vi "OutputSwerveAzimuth.vi"() -> ()   [LabVIEW 2020]
doc: "This VI runs feedback and feedforward controllers, manages safety interlocks, and sends commands to the swerve azimuth motors."
uses:
  robotoutputs.vi
  sensordata.vi
  TAI_Motor.vi
  <vilib>/Rock Robotics/WPI/ThirdParty/Phoenix-LabVIEW/Motor Controller/Controls/CTRE_Phoenix_MotorControl_ControlMode.ctl
  driverdata.vi
  <vilib>/Rock Robotics/WPI/ThirdParty/Phoenix-LabVIEW/Motor Controller/Controls/CTRE_Phoenix_MotorControl_NeutralMode.ctl
  6e813111-160f-47d9-be7e-04f12fb0a952.vi
  GRNF_CTREMotor.vi
  <vilib>/Rock Robotics/WPI/ThirdParty/Phoenix-LabVIEW/Motor Controller/Get/CTRE_Phoenix_MotorController_GetSelectedSensorData.vi
  GlobalDrivebase.vi
panel:
  in  "Slew Rate When Slow (/s)":dbl=50000.0
  in  "Slew Rate When Fast (/s)":dbl=5000.0
  out "Azimuth Error (deg)":dbl
  out "Azimuth Velocity":cluster{dbl}(graph)
  out "Azimuth Position":cluster{dbl, "Interlock Output":dbl}(graph)
  in  "PID Parameters":T1={"Kp"=0.3, "Ki"=0.0, "Kd"=0.0, "Kf (don't use)"=0.0, "I-Zone"=10.0} {"Kd" min=0.0; "Ki" min=0.0; "Kp" min=0.0}
  in  "Manual Azimuth Goal (deg) [-180,180]":dbl step=5.0
  in  "Manually Override Azimuth Goal":bool
  in  "Best Angle Hysteresis (deg)":dbl=20.0 format="%#_13g"
  in  "Plotting":T2(ring)
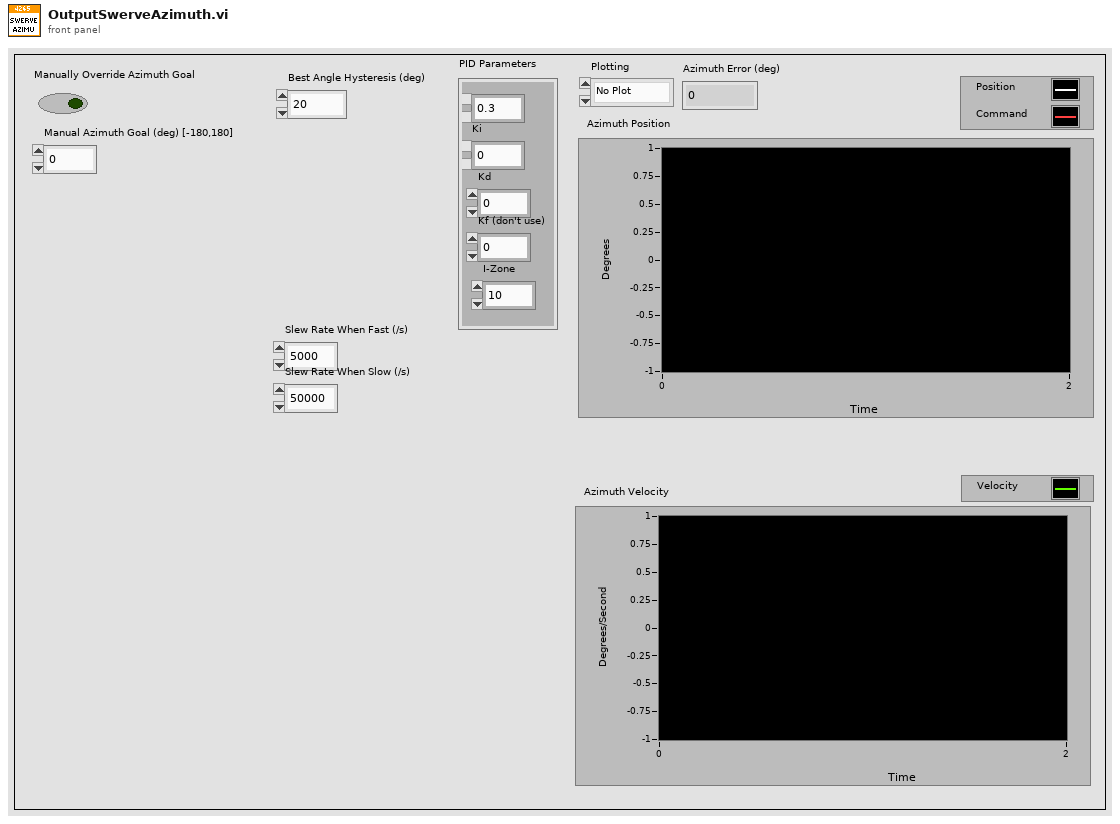
[diagram p1: front panel]
types:
  T1 = cluster{"Kp":dbl, "Ki":dbl, "Kd":dbl, "Kf (don't use)":dbl, "I-Zone":dbl}
  T2 = enum16{"No Plot", "Module 0", "Module 1", "Module 2", "Module 3"}
  T3 = cluster{"Kp":bool, "Ki":bool, "Kd":bool, "Kf (don't use)":bool, "I-Zone":bool}
  T4 = typedef "WPI_MotorControlDeviceRef.ctl" = cluster{"DeviceStatus":errorcluster, "Type":T5, "PWM":cluster{"PWM Channel":T6, "DeadBand":T7}, "CAN":cluster{"Device Number":u8, "SetOutput VI Ref":variant, "GetOutput VI Ref":variant, "Enable VI Ref":variant, "Disable VI Ref":variant, "Data":variant}, "Invert":bool, "DIO PWM":cluster{"PWM \"Enable\" Channel":T6, "DIOChannel":T8, "PWM Rate":dbl}}
  T5 = typedef "WPI_MotorControlType.ctl" = enum16{"PWM", "CAN", "DIO PWM"}
  T6 = typedef "FPGA_DIOPWMChannel.ctl" = enum8{"PWM 0", "PWM 1", "PWM 2", "PWM 3", "PWM 4", "PWM 5", "PWM 6", "PWM 7", "PWM 8", "PWM 9", "PWM MXP 0", "PWM MXP 1", "PWM MXP 2", "PWM MXP 3", "PWM MXP 4", "PWM MXP 5", "PWM MXP 6", "PWM MXP 7", "PWM MXP 8", "PWM MXP 9", "Invalid"}
  T7 = typedef "WPI_PWMDeadband.ctl" = cluster{"Name":string, "maxPositivePwm":i32, "minPositivePwm":i32, "centerPwm":i32, "maxNegativePwm":i32, "minNegativePwm":i32, "angularRange":u16}
  T8 = typedef "FPGA_DIOChannel.ctl" = enum8{"DIO 0", "DIO 1", "DIO 2", "DIO 3", "DIO 4", "DIO 5", "DIO 6", "DIO 7", "DIO 8", "DIO 9", "DIO MXP 0", "DIO MXP 1", "DIO MXP 2", "DIO MXP 3", "DIO MXP 4", "DIO MXP 5", "DIO MXP 6", "DIO MXP 7", "DIO MXP 8", "DIO MXP 9", "DIO MXP 10", "DIO MXP 11", "DIO MXP 12", "DIO MXP 13", "DIO MXP 14", "DIO MXP 15", "SPI Port CS1", "SPI Port CS2", "SPI Port CS3", "SPI Port MISO", "SPI Port MOSI", "Invalid"}
  T9 = typedef "CTRE_Phoenix_MotorControl_NeutralMode.ctl" = enum8{"EEPROMSetting", "Override to Coast", "Override to Brake"}
  T10 = typedef "CTRE_Phoenix_MotorControl_ControlMode.ctl" = u16
  T11 = enum16{"No Changed Output", "New Normal Output", "New Testing Output"}
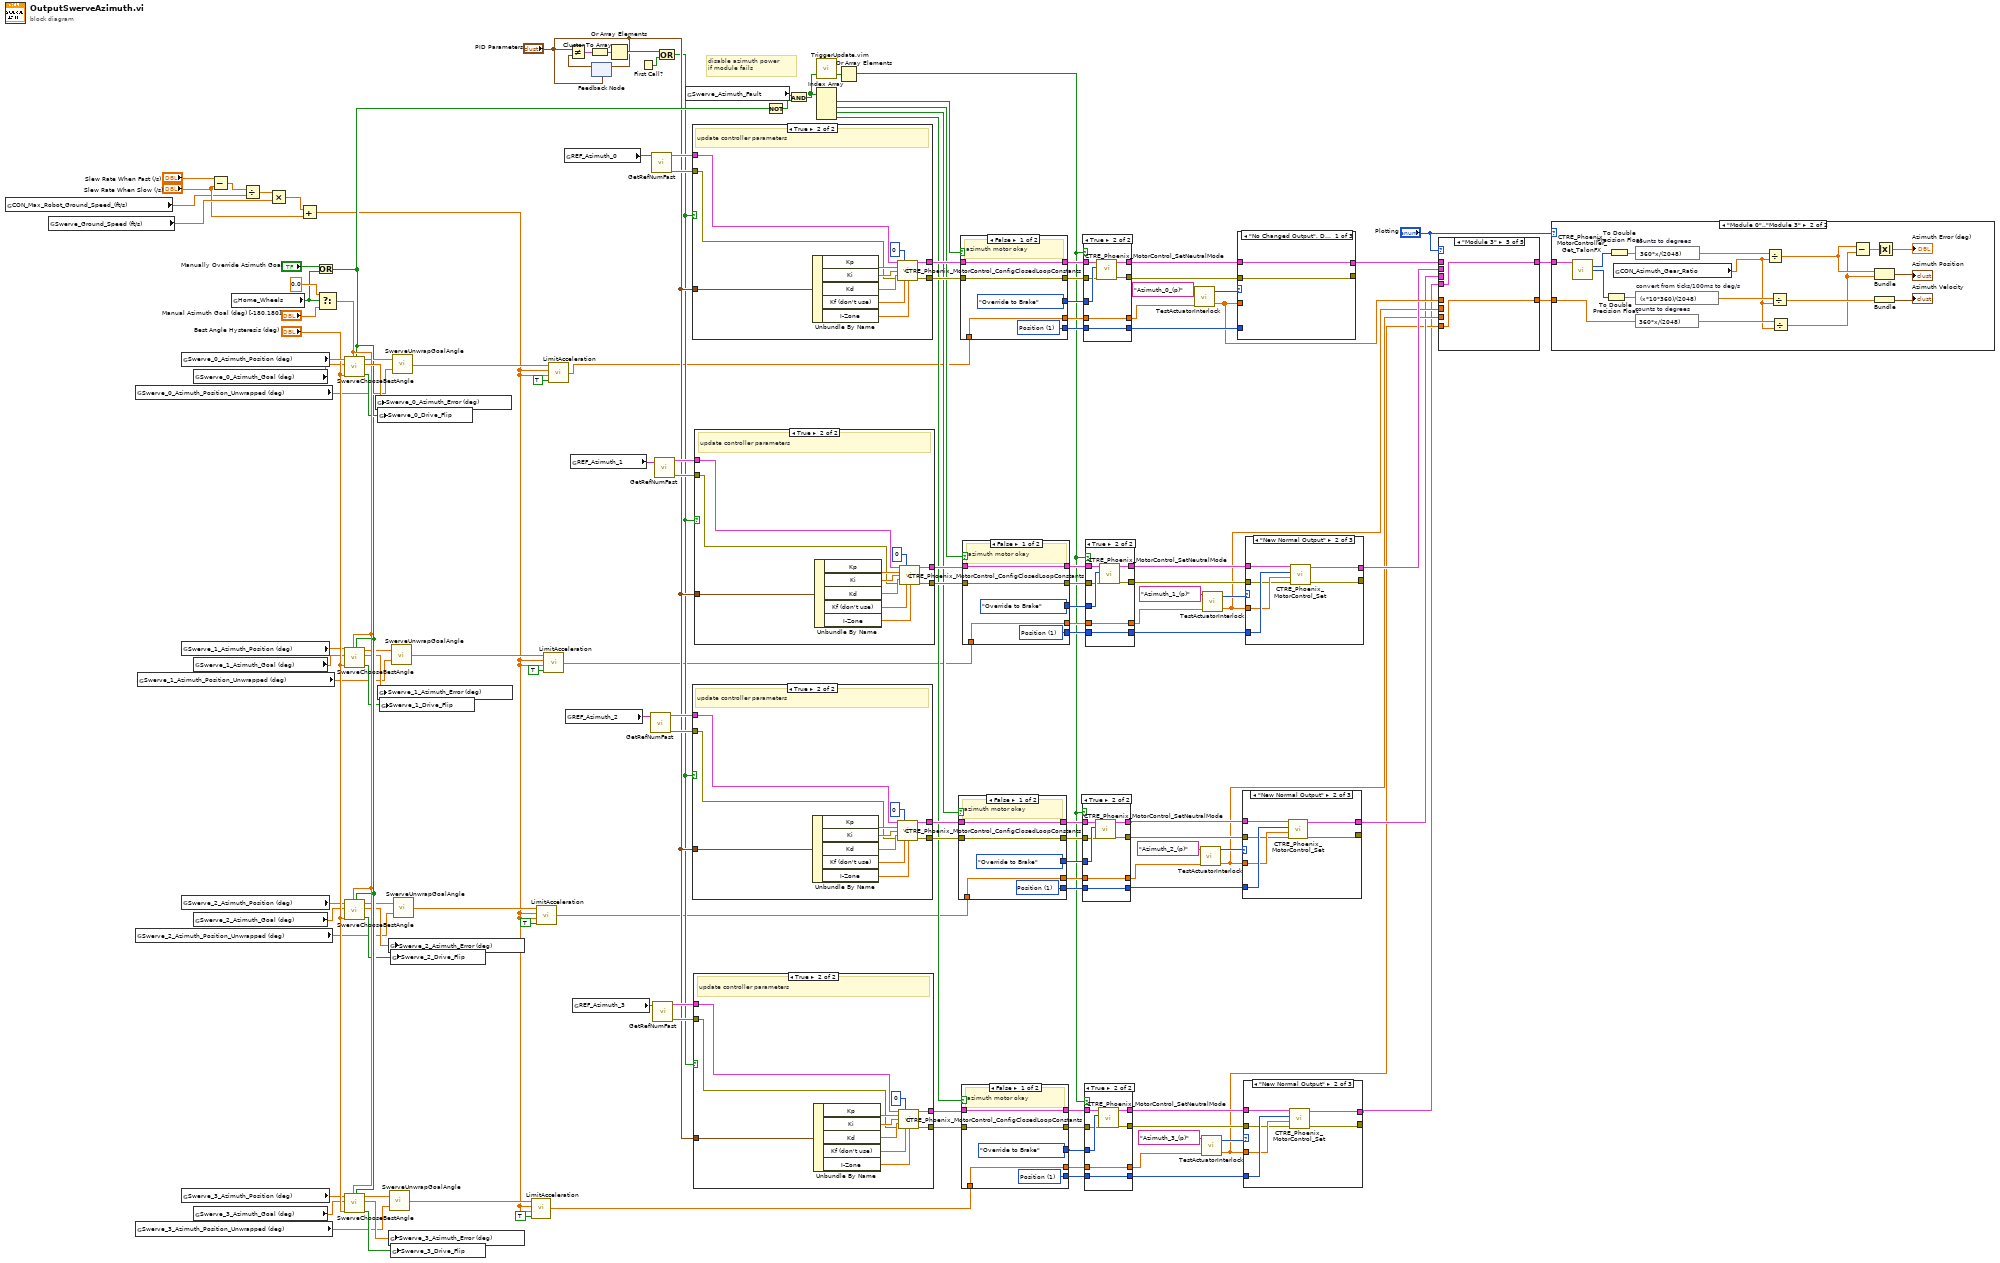
[diagram p0: block diagram]
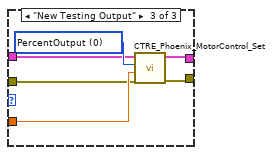
[diagram p3: hidden frame]
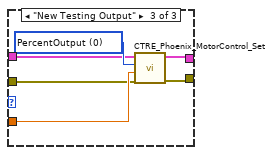
[diagram p5: hidden frame]
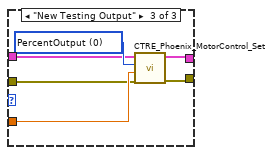
[diagram p7: hidden frame]
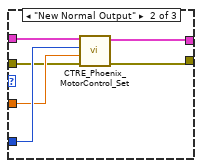
[diagram p8: hidden frame]
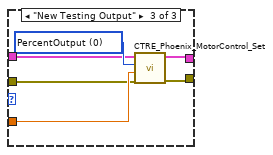
[diagram p9: hidden frame]
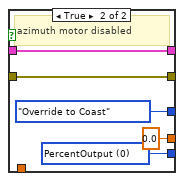
[diagram p12: hidden frame]
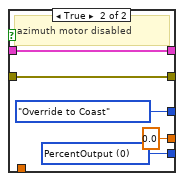
[diagram p15: hidden frame]
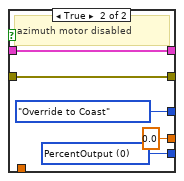
[diagram p18: hidden frame]
diagram:
  # "disable azimuth power\nif module fails"
  n1 = global read "GlobalDrivebase.vi" "CON_Max_Robot_Ground_Speed_(ft/s)"() -> (w1:dbl)
  n2 = global read "sensordata.vi" "Swerve_Ground_Speed (ft/s)"() -> (w9:dbl)
  n3 = global read "sensordata.vi" "Swerve_0_Azimuth_Position_Unwrapped (deg)"() -> (w113:dbl)
  n4 = global read "sensordata.vi" "Swerve_2_Azimuth_Position_Unwrapped (deg)"() -> (w26:dbl)
  n5 = global read "sensordata.vi" "Swerve_3_Azimuth_Position_Unwrapped (deg)"() -> (w24:dbl)
  n6 = global read "sensordata.vi" "Swerve_1_Azimuth_Position_Unwrapped (deg)"() -> (w28:dbl)
  n7 = global read "sensordata.vi" "Swerve_0_Azimuth_Position (deg)"() -> (w135:dbl)
  n8 = global read "sensordata.vi" "Swerve_1_Azimuth_Position (deg)"() -> (w37:dbl)
  n9 = global read "sensordata.vi" "Swerve_2_Azimuth_Position (deg)"() -> (w36:dbl)
  n10 = global read "sensordata.vi" "Swerve_3_Azimuth_Position (deg)"() -> (w35:dbl)
  n11 = global read "robotoutputs.vi" "Swerve_0_Azimuth_Goal (deg)"() -> (w5:dbl)
  n12 = global read "robotoutputs.vi" "Swerve_1_Azimuth_Goal (deg)"() -> (w34:dbl)
  n13 = global read "robotoutputs.vi" "Swerve_2_Azimuth_Goal (deg)"() -> (w33:dbl)
  n14 = global read "robotoutputs.vi" "Swerve_3_Azimuth_Goal (deg)"() -> (w32:dbl)
  n15 = Subtract(x="Slew Rate When Fast (/s)", y="Slew Rate When Slow (/s)") -> (x-y=w11:dbl)
  n16 = global read "driverdata.vi" "Home_Wheels"() -> (w137:bool)
  n17 = Divide(x=w11, y=w1) -> (x/y=w10:dbl)
  n18 = Multiply(x=w10, y=w9) -> (x*y=w7:dbl)
  n19 = Add(x=w7, y="Slew Rate When Slow (/s)") -> (x+y=w8:dbl)
  n20 = Or(x="Manually Override Azimuth Goal", y=w137) -> (x .or. y?=w109:bool)
  n21 = Select(t=0.0 ("f"), s=w137, f="Manual Azimuth Goal (deg) [-180,180]") -> (s? t:f=w134:dbl)
  n22 = call "SwerveChooseBestAngle.vi"("Goal Override"=w109, "Goal Override Angle (deg) [-180,+180]"=w134, "Hysteresis (deg)"="Best Angle Hysteresis (deg)", "Goal Angle (deg) [-180,+180]"=w5, "Current Angle (deg) [-180,+180]"=w135) -> ("Flip Drive Motor Direction"=w132:bool, "Flipped Angular Distance (deg)"=w136:dbl, "Flipped Goal Angle (deg) [-180, +180]"=w131:dbl)  [unwired: 4 in]
  n23 = call "SwerveChooseBestAngle.vi"("Goal Override"=w109, "Goal Override Angle (deg) [-180,+180]"=w134, "Hysteresis (deg)"="Best Angle Hysteresis (deg)", "Goal Angle (deg) [-180,+180]"=w34, "Current Angle (deg) [-180,+180]"=w37) -> ("Flip Drive Motor Direction"=w31:bool, "Flipped Angular Distance (deg)"=w40:dbl, "Flipped Goal Angle (deg) [-180, +180]"=w27:dbl)  [unwired: 4 in]
  n24 = call "SwerveChooseBestAngle.vi"("Goal Override"=w109, "Goal Override Angle (deg) [-180,+180]"=w134, "Hysteresis (deg)"="Best Angle Hysteresis (deg)", "Goal Angle (deg) [-180,+180]"=w33, "Current Angle (deg) [-180,+180]"=w36) -> ("Flip Drive Motor Direction"=w30:bool, "Flipped Angular Distance (deg)"=w39:dbl, "Flipped Goal Angle (deg) [-180, +180]"=w25:dbl)  [unwired: 4 in]
  n25 = call "SwerveChooseBestAngle.vi"("Goal Override"=w109, "Goal Override Angle (deg) [-180,+180]"=w134, "Hysteresis (deg)"="Best Angle Hysteresis (deg)", "Goal Angle (deg) [-180,+180]"=w32, "Current Angle (deg) [-180,+180]"=w35) -> ("Flip Drive Motor Direction"=w29:bool, "Flipped Angular Distance (deg)"=w38:dbl, "Flipped Goal Angle (deg) [-180, +180]"=w23:dbl)  [unwired: 4 in]
  n26 = global write "robotoutputs.vi" "Swerve_0_Azimuth_Error (deg)"(w136) -> ()
  n27 = global write "robotoutputs.vi" "Swerve_1_Azimuth_Error (deg)"(w40) -> ()
  n28 = global write "robotoutputs.vi" "Swerve_0_Drive_Flip"(w132) -> ()
  n29 = global write "robotoutputs.vi" "Swerve_1_Drive_Flip"(w31) -> ()
  n30 = global write "robotoutputs.vi" "Swerve_2_Azimuth_Error (deg)"(w39) -> ()
  n31 = global write "robotoutputs.vi" "Swerve_3_Azimuth_Error (deg)"(w38) -> ()
  n32 = call "SwerveUnwrapGoalAngle.vi"("Current Unwrapped Angle (deg) [-Inf,+Inf]"=w24, "Flipped Goal Angle (deg) [-180, +180]"=w23) -> ("Absolute Azimuth Position (tics) [-Inf,+Inf]"=w16:dbl)
  n33 = global write "robotoutputs.vi" "Swerve_2_Drive_Flip"(w30) -> ()
  n34 = global write "robotoutputs.vi" "Swerve_3_Drive_Flip"(w29) -> ()
  n35 = call "SwerveUnwrapGoalAngle.vi"("Current Unwrapped Angle (deg) [-Inf,+Inf]"=w28, "Flipped Goal Angle (deg) [-180, +180]"=w27) -> ("Absolute Azimuth Position (tics) [-Inf,+Inf]"=w22:dbl)
  n36 = call "SwerveUnwrapGoalAngle.vi"("Current Unwrapped Angle (deg) [-Inf,+Inf]"=w113, "Flipped Goal Angle (deg) [-180, +180]"=w131) -> ("Absolute Azimuth Position (tics) [-Inf,+Inf]"=w41:dbl)
  n37 = call "SwerveUnwrapGoalAngle.vi"("Current Unwrapped Angle (deg) [-Inf,+Inf]"=w26, "Flipped Goal Angle (deg) [-180, +180]"=w25) -> ("Absolute Azimuth Position (tics) [-Inf,+Inf]"=w18:dbl)
  n38 = call "LimitAcceleration.vi"("Apply Limit"=TRUE, "Decceleration Limit (/s)"=w8, "Acceleration Limit (/s)"=w8, "Raw Input"=w16) -> ("Output"=w13:dbl)
  n39 = call "LimitAcceleration.vi"("Apply Limit"=TRUE, "Decceleration Limit (/s)"=w8, "Acceleration Limit (/s)"=w8, "Raw Input"=w18) -> ("Output"=w17:dbl)
  n40 = call "LimitAcceleration.vi"("Apply Limit"=TRUE, "Decceleration Limit (/s)"=w8, "Acceleration Limit (/s)"=w8, "Raw Input"=w22) -> ("Output"=w19:dbl)
  n41 = call "LimitAcceleration.vi"("Apply Limit"=TRUE, "Decceleration Limit (/s)"=w8, "Acceleration Limit (/s)"=w8, "Raw Input"=w41) -> ("Output"=w42:dbl)
  n42 = global read "GlobalDrivebase.vi" "REF_Azimuth_0"() -> (w141:string)
  n43 = global read "GlobalDrivebase.vi" "REF_Azimuth_2"() -> (w3:string)
  n44 = global read "GlobalDrivebase.vi" "REF_Azimuth_1"() -> (w4:string)
  n45 = global read "GlobalDrivebase.vi" "REF_Azimuth_3"() -> (w2:string)
  n46 = feedback #1("PID Parameters") -> (w128:T1)
  n47 = Not Equal?(x="PID Parameters", y=w128) -> (x != y?=w130:T3)
  n48 = Cluster To Array(cluster=w130) -> (array=w129:bool[])
  n49 = feedback-in #1("PID Parameters") -> ()
  n50 = Or Array Elements(Boolean array=w129) -> (logical OR=w127:bool)
  n51 = First Call?() -> (First Call?: T/F=w126:bool)
  n52 = call-poly "GetRefNumFast.vi"("RefNum Name"=w3) -> ("Error"=w97:errorcluster, "Device Reference"=w98:T4)  [unwired: 5 in]
  n53 = call-poly "GetRefNumFast.vi"("RefNum Name"=w141) -> ("Error"=w124:errorcluster, "Device Reference"=w125:T4)  [unwired: 5 in]
  n54 = call-poly "GetRefNumFast.vi"("RefNum Name"=w2) -> ("Error"=w87:errorcluster, "Device Reference"=w88:T4)  [unwired: 5 in]
  n55 = call-poly "GetRefNumFast.vi"("RefNum Name"=w4) -> ("Error"=w107:errorcluster, "Device Reference"=w108:T4)  [unwired: 5 in]
  n56 = Compound Arithmetic op=OR(w127, w126) -> (w78:bool)
  n57 = global read "sensordata.vi" "Swerve_Azimuth_Fault"() -> (w112:bool[])
  n58 = case shown="True" w78 {
    tunnel: "PID Parameters" -> [_ w151]
    tunnel: [w144 w148] -> w123
    tunnel: [w143 w147] -> w122
    tunnel: w125 -> [w144 w146]
    tunnel: w124 -> [w143 w145]
    frame False {
      # "holde controller parameters"
    }
    frame True {
      # "update controller parameters"
      n59 = Unbundle By Name(w151) -> ("Kp"=w155:dbl, "Ki"=w154:dbl, "Kd"=w153:dbl, "Kf (don't use)"=w150:dbl, "I-Zone"=w149:dbl)
      n60 = call <vilib>:"CTRE_Phoenix_MotorControl_ConfigClosedLoopConstants.vi"("PhoenixMotorControlDevRef"=w146, "slotIdx"=0, "P"=w155, "I"=w154, "D"=w153, "error in (no error)"=w145, "F"=w150, "I Zone"=w149) -> ("PhoenixMotorControlDevRef"=w148:T4, "error out"=w147:errorcluster)  [unwired: 6 in]
    }
  }
  n61 = case shown="True" w78 {
    tunnel: "PID Parameters" -> [_ w164]
    tunnel: [w157 w161] -> w96
    tunnel: [w156 w160] -> w95
    tunnel: w98 -> [w157 w159]
    tunnel: w97 -> [w156 w158]
    frame False {
      # "holde controller parameters"
    }
    frame True {
      # "update controller parameters"
      n62 = Unbundle By Name(w164) -> ("Kp"=w168:dbl, "Ki"=w167:dbl, "Kd"=w166:dbl, "Kf (don't use)"=w163:dbl, "I-Zone"=w162:dbl)
      n63 = call <vilib>:"CTRE_Phoenix_MotorControl_ConfigClosedLoopConstants.vi"("PhoenixMotorControlDevRef"=w159, "slotIdx"=0, "P"=w168, "I"=w167, "D"=w166, "error in (no error)"=w158, "F"=w163, "I Zone"=w162) -> ("PhoenixMotorControlDevRef"=w161:T4, "error out"=w160:errorcluster)  [unwired: 6 in]
    }
  }
  n64 = case shown="True" w78 {
    tunnel: "PID Parameters" -> [_ w177]
    tunnel: [w170 w174] -> w86
    tunnel: [w169 w173] -> w85
    tunnel: w88 -> [w170 w172]
    tunnel: w87 -> [w169 w171]
    frame False {
      # "holde controller parameters"
    }
    frame True {
      # "update controller parameters"
      n65 = Unbundle By Name(w177) -> ("Kp"=w181:dbl, "Ki"=w180:dbl, "Kd"=w179:dbl, "Kf (don't use)"=w176:dbl, "I-Zone"=w175:dbl)
      n66 = call <vilib>:"CTRE_Phoenix_MotorControl_ConfigClosedLoopConstants.vi"("PhoenixMotorControlDevRef"=w172, "slotIdx"=0, "P"=w181, "I"=w180, "D"=w179, "error in (no error)"=w171, "F"=w176, "I Zone"=w175) -> ("PhoenixMotorControlDevRef"=w174:T4, "error out"=w173:errorcluster)  [unwired: 6 in]
    }
  }
  n67 = case shown="True" w78 {
    tunnel: "PID Parameters" -> [_ w190]
    tunnel: [w183 w187] -> w106
    tunnel: [w182 w186] -> w105
    tunnel: w108 -> [w183 w185]
    tunnel: w107 -> [w182 w184]
    frame False {
      # "holde controller parameters"
    }
    frame True {
      # "update controller parameters"
      n68 = Unbundle By Name(w190) -> ("Kp"=w194:dbl, "Ki"=w193:dbl, "Kd"=w192:dbl, "Kf (don't use)"=w189:dbl, "I-Zone"=w188:dbl)
      n69 = call <vilib>:"CTRE_Phoenix_MotorControl_ConfigClosedLoopConstants.vi"("PhoenixMotorControlDevRef"=w185, "slotIdx"=0, "P"=w194, "I"=w193, "D"=w192, "error in (no error)"=w184, "F"=w189, "I Zone"=w188) -> ("PhoenixMotorControlDevRef"=w187:T4, "error out"=w186:errorcluster)  [unwired: 6 in]
    }
  }
  n70 = Not(x=w109) -> (.not. x?=w110:bool)
  n71 = And(x=w112, y=w110) -> (x .and. y?=w111:bool[])
  n72 = call "TriggerUpdate.vim"("Trigger"=w111) -> ("Update"=w118:bool[])  [unwired: 2 in]
  n73 = Index Array(array=w111) -> (element #1=w142:bool, element #2=w99:bool, element #3=w89:bool, element #4=w77:bool)  [unwired: 4 in]
  n74 = Or Array Elements(Boolean array=w118) -> (logical OR=w76:bool)
  n75 = case shown="False" w89 {
    tunnel: [w199 w204] -> w93
    tunnel: w96 -> [w199 w204]
    tunnel: [w195 0.0 ("Command")] -> w91
    tunnel: [w198 w202] -> w90
    tunnel: [CTRE_Phoenix_MotorControl_NeutralMode."Override to Brake" ("Motor Control Neutral Mode") CTRE_Phoenix_MotorControl_NeutralMode."Override to Coast" ("Motor Control Neutral Mode")] -> w94
    tunnel: w95 -> [w196 w200]
    tunnel: [w196 w200] -> w92
    tunnel: w17 -> [w195 _]
    frame False {
      w198 = T10 1 items=["PercentOutput"=0, "Position"=1, "Velocity"=2, "Current"=3, "Follower"=5, "MotionProfile"=6, "MotionMagic"=7, "MotionProfileArc"=10, "Disabled"=15] ("Control Mode")
      # "azimuth motor okay"
    }
    frame True {
      w202 = T10 0 items=["PercentOutput"=0, "Position"=1, "Velocity"=2, "Current"=3, "Follower"=5, "MotionProfile"=6, "MotionMagic"=7, "MotionProfileArc"=10, "Disabled"=15] ("Control Mode")
      # "azimuth motor disabled"
    }
  }
  n76 = case shown="False" w142 {
    tunnel: [w209 w214] -> w120
    tunnel: w123 -> [w209 w214]
    tunnel: [w205 0.0 ("Command")] -> w117
    tunnel: [w208 w212] -> w116
    tunnel: [CTRE_Phoenix_MotorControl_NeutralMode."Override to Brake" ("Motor Control Neutral Mode") CTRE_Phoenix_MotorControl_NeutralMode."Override to Coast" ("Motor Control Neutral Mode")] -> w121
    tunnel: w122 -> [w206 w210]
    tunnel: [w206 w210] -> w119
    tunnel: w42 -> [w205 _]
    frame False {
      w208 = T10 1 items=["PercentOutput"=0, "Position"=1, "Velocity"=2, "Current"=3, "Follower"=5, "MotionProfile"=6, "MotionMagic"=7, "MotionProfileArc"=10, "Disabled"=15] ("Control Mode")
      # "azimuth motor okay"
    }
    frame True {
      w212 = T10 0 items=["PercentOutput"=0, "Position"=1, "Velocity"=2, "Current"=3, "Follower"=5, "MotionProfile"=6, "MotionMagic"=7, "MotionProfileArc"=10, "Disabled"=15] ("Control Mode")
      # "azimuth motor disabled"
    }
  }
  n77 = case shown="False" w77 {
    tunnel: [w219 w224] -> w83
    tunnel: w86 -> [w219 w224]
    tunnel: [w215 0.0 ("Command")] -> w81
    tunnel: [w218 w222] -> w80
    tunnel: [CTRE_Phoenix_MotorControl_NeutralMode."Override to Brake" ("Motor Control Neutral Mode") CTRE_Phoenix_MotorControl_NeutralMode."Override to Coast" ("Motor Control Neutral Mode")] -> w84
    tunnel: w85 -> [w216 w220]
    tunnel: [w216 w220] -> w82
    tunnel: w13 -> [w215 _]
    frame False {
      w218 = T10 1 items=["PercentOutput"=0, "Position"=1, "Velocity"=2, "Current"=3, "Follower"=5, "MotionProfile"=6, "MotionMagic"=7, "MotionProfileArc"=10, "Disabled"=15] ("Control Mode")
      # "azimuth motor okay"
    }
    frame True {
      w222 = T10 0 items=["PercentOutput"=0, "Position"=1, "Velocity"=2, "Current"=3, "Follower"=5, "MotionProfile"=6, "MotionMagic"=7, "MotionProfileArc"=10, "Disabled"=15] ("Control Mode")
      # "azimuth motor disabled"
    }
  }
  n78 = case shown="False" w99 {
    tunnel: [w229 w234] -> w103
    tunnel: w106 -> [w229 w234]
    tunnel: [w225 0.0 ("Command")] -> w101
    tunnel: [w228 w232] -> w100
    tunnel: [CTRE_Phoenix_MotorControl_NeutralMode."Override to Brake" ("Motor Control Neutral Mode") CTRE_Phoenix_MotorControl_NeutralMode."Override to Coast" ("Motor Control Neutral Mode")] -> w104
    tunnel: w105 -> [w226 w230]
    tunnel: [w226 w230] -> w102
    tunnel: w19 -> [w225 _]
    frame False {
      w228 = T10 1 items=["PercentOutput"=0, "Position"=1, "Velocity"=2, "Current"=3, "Follower"=5, "MotionProfile"=6, "MotionMagic"=7, "MotionProfileArc"=10, "Disabled"=15] ("Control Mode")
      # "azimuth motor okay"
    }
    frame True {
      w232 = T10 0 items=["PercentOutput"=0, "Position"=1, "Velocity"=2, "Current"=3, "Follower"=5, "MotionProfile"=6, "MotionMagic"=7, "MotionProfileArc"=10, "Disabled"=15] ("Control Mode")
      # "azimuth motor disabled"
    }
  }
  n79 = case shown="True" w76 {
    tunnel: w94 -> [_ w245]
    tunnel: w93 -> [w238 w244]
    tunnel: w92 -> [w237 w243]
    tunnel: [w238 w242] -> w57
    tunnel: [w237 w241] -> w56
    tunnel: w91 -> [w236 w240]
    tunnel: [w236 w240] -> w55
    tunnel: w90 -> [w235 w239]
    tunnel: [w235 w239] -> w54
    frame False {
    }
    frame True {
      n80 = call <vilib>:"CTRE_Phoenix_MotorControl_SetNeutralMode.vi"("error in (no error)"=w243, "Motor Control Neutral Mode"=w245, "PhoenixMotorControlDevRef"=w244) -> ("error out"=w241:errorcluster, "PhoenixMotorControlDevRef"=w242:T4)  [unwired: 7 in]
    }
  }
  n81 = case shown="True" w76 {
    tunnel: w121 -> [_ w256]
    tunnel: w120 -> [w249 w255]
    tunnel: w119 -> [w248 w254]
    tunnel: [w249 w253] -> w73
    tunnel: [w248 w252] -> w72
    tunnel: w117 -> [w247 w251]
    tunnel: [w247 w251] -> w70
    tunnel: w116 -> [w246 w250]
    tunnel: [w246 w250] -> w71
    frame False {
    }
    frame True {
      n82 = call <vilib>:"CTRE_Phoenix_MotorControl_SetNeutralMode.vi"("error in (no error)"=w254, "Motor Control Neutral Mode"=w256, "PhoenixMotorControlDevRef"=w255) -> ("error out"=w252:errorcluster, "PhoenixMotorControlDevRef"=w253:T4)  [unwired: 7 in]
    }
  }
  n83 = case shown="True" w76 {
    tunnel: w84 -> [_ w267]
    tunnel: w83 -> [w260 w266]
    tunnel: w82 -> [w259 w265]
    tunnel: [w260 w264] -> w49
    tunnel: [w259 w263] -> w48
    tunnel: w81 -> [w258 w262]
    tunnel: [w258 w262] -> w47
    tunnel: w80 -> [w257 w261]
    tunnel: [w257 w261] -> w46
    frame False {
    }
    frame True {
      n84 = call <vilib>:"CTRE_Phoenix_MotorControl_SetNeutralMode.vi"("error in (no error)"=w265, "Motor Control Neutral Mode"=w267, "PhoenixMotorControlDevRef"=w266) -> ("error out"=w263:errorcluster, "PhoenixMotorControlDevRef"=w264:T4)  [unwired: 7 in]
    }
  }
  n85 = case shown="True" w76 {
    tunnel: w104 -> [_ w278]
    tunnel: w103 -> [w271 w277]
    tunnel: w102 -> [w270 w276]
    tunnel: [w271 w275] -> w62
    tunnel: [w270 w274] -> w63
    tunnel: w101 -> [w269 w273]
    tunnel: [w269 w273] -> w64
    tunnel: w100 -> [w268 w272]
    tunnel: [w268 w272] -> w65
    frame False {
    }
    frame True {
      n86 = call <vilib>:"CTRE_Phoenix_MotorControl_SetNeutralMode.vi"("error in (no error)"=w276, "Motor Control Neutral Mode"=w278, "PhoenixMotorControlDevRef"=w277) -> ("error out"=w274:errorcluster, "PhoenixMotorControlDevRef"=w275:T4)  [unwired: 7 in]
    }
  }
  n87 = call-poly "TestActuatorInterlock.vi"("Normal Output"=w70, "Actuator Name"="Azimuth_0_(p)" ("Actuator_Name")) -> ("Interlocked Output"=w69:dbl, "Output Mode"=w75:T11)  [unwired: 3 in]
  n88 = call-poly "TestActuatorInterlock.vi"("Normal Output"=w55, "Actuator Name"="Azimuth_2_(p)" ("Actuator_Name")) -> ("Interlocked Output"=w53:dbl, "Output Mode"=w59:T11)  [unwired: 3 in]
  n89 = call-poly "TestActuatorInterlock.vi"("Normal Output"=w47, "Actuator Name"="Azimuth_3_(p)" ("Actuator_Name")) -> ("Interlocked Output"=w45:dbl, "Output Mode"=w51:T11)  [unwired: 3 in]
  n90 = call-poly "TestActuatorInterlock.vi"("Normal Output"=w64, "Actuator Name"="Azimuth_1_(p)" ("Actuator_Name")) -> ("Interlocked Output"=w60:dbl, "Output Mode"=w67:T11)  [unwired: 3 in]
  n91 = case shown="\"No Changed Output\", Default" w75 {
    tunnel: w71 -> [_ w286 _]
    tunnel: w73 -> [w280 w284 w291]
    tunnel: w69 -> [_ w285 w290]
    tunnel: w72 -> [w279 w281 w289]
    tunnel: [w280 w283 w288] -> w68
    tunnel: [w279 w282 w287] -> _
    frame "No Changed Output", Default {
    }
    frame "New Normal Output" {
      n92 = call <vilib>:"CTRE_Phoenix_MotorControl_Set.vi"("error in (no error)"=w281, "Output"=w285, "Control Mode"=w286, "PhoenixMotorControlDevRef"=w284) -> ("error out"=w282:errorcluster, "PhoenixMotorControlDevRef"=w283:T4)  [unwired: 6 in]
    }
    frame "New Testing Output" {
      w292 = T10 0 items=["PercentOutput"=0, "Position"=1, "Velocity"=2, "Current"=3, "Follower"=5, "MotionProfile"=6, "MotionMagic"=7, "MotionProfileArc"=10, "Disabled"=15] ("Control Mode")
      n93 = call <vilib>:"CTRE_Phoenix_MotorControl_Set.vi"("error in (no error)"=w289, "Output"=w290, "Control Mode"=w292, "PhoenixMotorControlDevRef"=w291) -> ("error out"=w287:errorcluster, "PhoenixMotorControlDevRef"=w288:T4)  [unwired: 6 in]
    }
  }
  n94 = case shown="\"New Normal Output\"" w59 {
    tunnel: w54 -> [_ w300 _]
    tunnel: w57 -> [w294 w298 w305]
    tunnel: w53 -> [_ w299 w304]
    tunnel: w56 -> [w293 w295 w303]
    tunnel: [w294 w297 w302] -> w52
    tunnel: [w293 w296 w301] -> _
    frame "No Changed Output", Default {
    }
    frame "New Normal Output" {
      n95 = call <vilib>:"CTRE_Phoenix_MotorControl_Set.vi"("error in (no error)"=w295, "Output"=w299, "Control Mode"=w300, "PhoenixMotorControlDevRef"=w298) -> ("error out"=w296:errorcluster, "PhoenixMotorControlDevRef"=w297:T4)  [unwired: 6 in]
    }
    frame "New Testing Output" {
      w306 = T10 0 items=["PercentOutput"=0, "Position"=1, "Velocity"=2, "Current"=3, "Follower"=5, "MotionProfile"=6, "MotionMagic"=7, "MotionProfileArc"=10, "Disabled"=15] ("Control Mode")
      n96 = call <vilib>:"CTRE_Phoenix_MotorControl_Set.vi"("error in (no error)"=w303, "Output"=w304, "Control Mode"=w306, "PhoenixMotorControlDevRef"=w305) -> ("error out"=w301:errorcluster, "PhoenixMotorControlDevRef"=w302:T4)  [unwired: 6 in]
    }
  }
  n97 = case shown="\"New Normal Output\"" w51 {
    tunnel: w46 -> [_ w314 _]
    tunnel: w49 -> [w308 w312 w319]
    tunnel: w45 -> [_ w313 w318]
    tunnel: w48 -> [w307 w309 w317]
    tunnel: [w308 w311 w316] -> w44
    tunnel: [w307 w310 w315] -> _
    frame "No Changed Output", Default {
    }
    frame "New Normal Output" {
      n98 = call <vilib>:"CTRE_Phoenix_MotorControl_Set.vi"("error in (no error)"=w309, "Output"=w313, "Control Mode"=w314, "PhoenixMotorControlDevRef"=w312) -> ("error out"=w310:errorcluster, "PhoenixMotorControlDevRef"=w311:T4)  [unwired: 6 in]
    }
    frame "New Testing Output" {
      w320 = T10 0 items=["PercentOutput"=0, "Position"=1, "Velocity"=2, "Current"=3, "Follower"=5, "MotionProfile"=6, "MotionMagic"=7, "MotionProfileArc"=10, "Disabled"=15] ("Control Mode")
      n99 = call <vilib>:"CTRE_Phoenix_MotorControl_Set.vi"("error in (no error)"=w317, "Output"=w318, "Control Mode"=w320, "PhoenixMotorControlDevRef"=w319) -> ("error out"=w315:errorcluster, "PhoenixMotorControlDevRef"=w316:T4)  [unwired: 6 in]
    }
  }
  n100 = case shown="\"New Normal Output\"" w67 {
    tunnel: w65 -> [_ w328 _]
    tunnel: w62 -> [w322 w326 w333]
    tunnel: w60 -> [_ w327 w332]
    tunnel: w63 -> [w321 w323 w331]
    tunnel: [w322 w325 w330] -> w61
    tunnel: [w321 w324 w329] -> _
    frame "No Changed Output", Default {
    }
    frame "New Normal Output" {
      n101 = call <vilib>:"CTRE_Phoenix_MotorControl_Set.vi"("error in (no error)"=w323, "Output"=w327, "Control Mode"=w328, "PhoenixMotorControlDevRef"=w326) -> ("error out"=w324:errorcluster, "PhoenixMotorControlDevRef"=w325:T4)  [unwired: 6 in]
    }
    frame "New Testing Output" {
      w334 = T10 0 items=["PercentOutput"=0, "Position"=1, "Velocity"=2, "Current"=3, "Follower"=5, "MotionProfile"=6, "MotionMagic"=7, "MotionProfileArc"=10, "Disabled"=15] ("Control Mode")
      n102 = call <vilib>:"CTRE_Phoenix_MotorControl_Set.vi"("error in (no error)"=w331, "Output"=w332, "Control Mode"=w334, "PhoenixMotorControlDevRef"=w333) -> ("error out"=w329:errorcluster, "PhoenixMotorControlDevRef"=w330:T4)  [unwired: 6 in]
    }
  }
  n103 = case shown="\"Module 3\"" "Plotting" {
    tunnel: w69 -> [_ w338 _ _ _]
    tunnel: [0.0 ("Interlock Output") w338 w340 w342 w344] -> w115
    tunnel: w68 -> [w335 w337 _ _ _]
    tunnel: [w335 w337 w339 w341 w343] -> w114
    tunnel: w60 -> [_ _ w340 _ _]
    tunnel: w61 -> [_ _ w339 _ _]
    tunnel: w53 -> [_ _ _ w342 _]
    tunnel: w52 -> [_ _ _ w341 _]
    tunnel: w45 -> [_ _ _ _ w344]
    tunnel: w44 -> [_ _ _ _ w343]
    frame "No Plot", Default {
    }
    frame "Module 0" {
    }
    frame "Module 1" {
    }
    frame "Module 2" {
    }
    frame "Module 3" {
    }
  }
  n104 = case shown="\"Module 0\"..\"Module 3\"" "Plotting" {
    tunnel: w115 -> [_ w355]
    tunnel: w114 -> [_ w356]
    frame "No Plot", Default {
    }
    frame "Module 0".."Module 3" {
      n105 = call-poly <vilib>:"CTRE_Phoenix_MotorController_Get_TalonFX.vi"("PhoenixMotorControlDevRef"=w356) -> ("Position (Raw Sensor Units)"=w360:i32, "Velocity (Raw Sensor Units per 100 ms)"=w359:i32)  [unwired: 11 in, 2 out]
      n106 = To Double Precision Float(number=w359) -> (double precision float=w358:dbl)
      n107 = To Double Precision Float(number=w360) -> (double precision float=w361:dbl)
      n108 = global read "GlobalDrivebase.vi" "CON_Azimuth_Gear_Ratio"() -> (w345:dbl)
      n109 = expression code="360*x/(2048)" "counts to degrees"(w355) -> (w347:dbl)
      n110 = expression code="360*x/(2048)" "counts to degrees"(w361) -> (w351:dbl)
      n111 = expression code="(x*10*360)/(2048)" "convert from ticks/100ms to deg/s"(w358) -> (w349:dbl)
      n112 = Divide(x=w351, y=w345) -> (x/y=w350:dbl)
      n113 = Divide(x=w349, y=w345) -> (x/y=w348:dbl)
      n114 = Divide(x=w347, y=w345) -> (x/y=w346:dbl)
      n115 = Subtract(x=w350, y=w346) -> (x-y=w353:dbl)
      n116 = Bundle(w350, w346) -> (→"Azimuth Position":cluster{dbl, dbl})  [unwired: 1 in]
      n117 = Bundle(w348) -> (→"Azimuth Velocity":cluster{dbl})  [unwired: 1 in]
      n118 = Absolute Value(x=w353) -> (abs(x)=→"Azimuth Error (deg)":dbl)
    }
  }
